vi "GetIQ.vi"(4 "contSwitch":dbl, 5 "solotSwitch":dbl, 6 "packSize":dbl, 7 "packNum":dbl, 8 "error in (no error)":errorcluster caption="错误输入（无错误）", 9 "freqDiv":dbl, 10 "soltNo":dbl, 11 "Path":path) -> (0 "error out":errorcluster caption="错误输出", 3 "getIQ":u8)   [LabVIEW 2015]
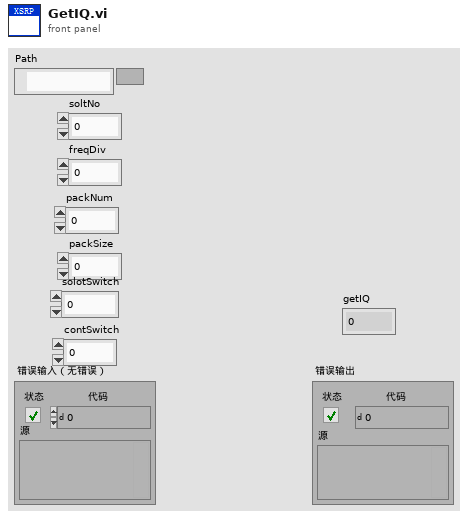
[diagram p1: front panel]
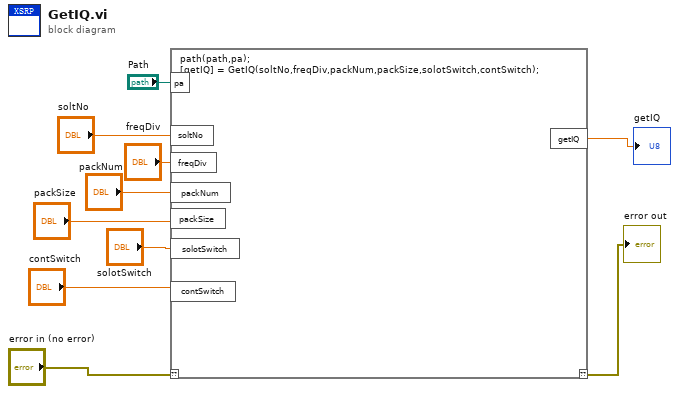
[diagram p0: block diagram]
diagram:
  n1 = script code="path(path,pa);\n[getIQ] = GetIQ(soltNo,freqDiv,packNum,packSize,solotSwitch,contSwitch);"("??"="error in (no error)", "pa"="Path", "soltNo"="soltNo", "freqDiv"="freqDiv", "packNum"="packNum", "packSize"="packSize", "solotSwitch"="solotSwitch", "contSwitch"="contSwitch") -> ("??"=→"error out":errorcluster, "getIQ"=→"getIQ":dbl)
